vi "BinAvgSub3.vi"(6 "X ref array":dbl[](array[numeric]), 7 "Extend to 0":bool, 9 "Bin size":dbl, 10 "X coumn index":i32, 11 "Data in":dbl[][](array[numeric])) -> (3 "Binned data":dbl[][](array[numeric]) format="%#_10g")   [LabVIEW 2018]
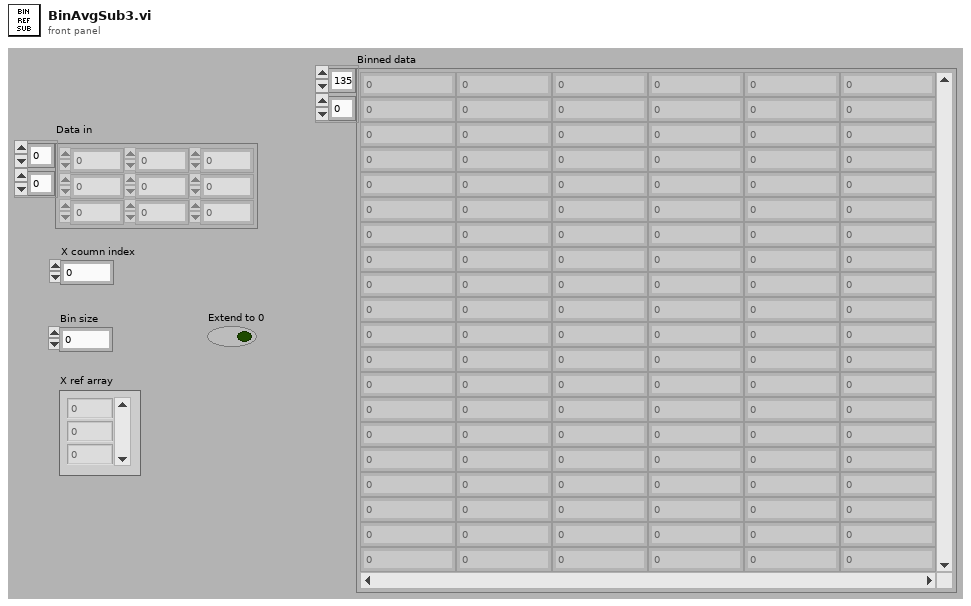
[diagram p1: front panel]
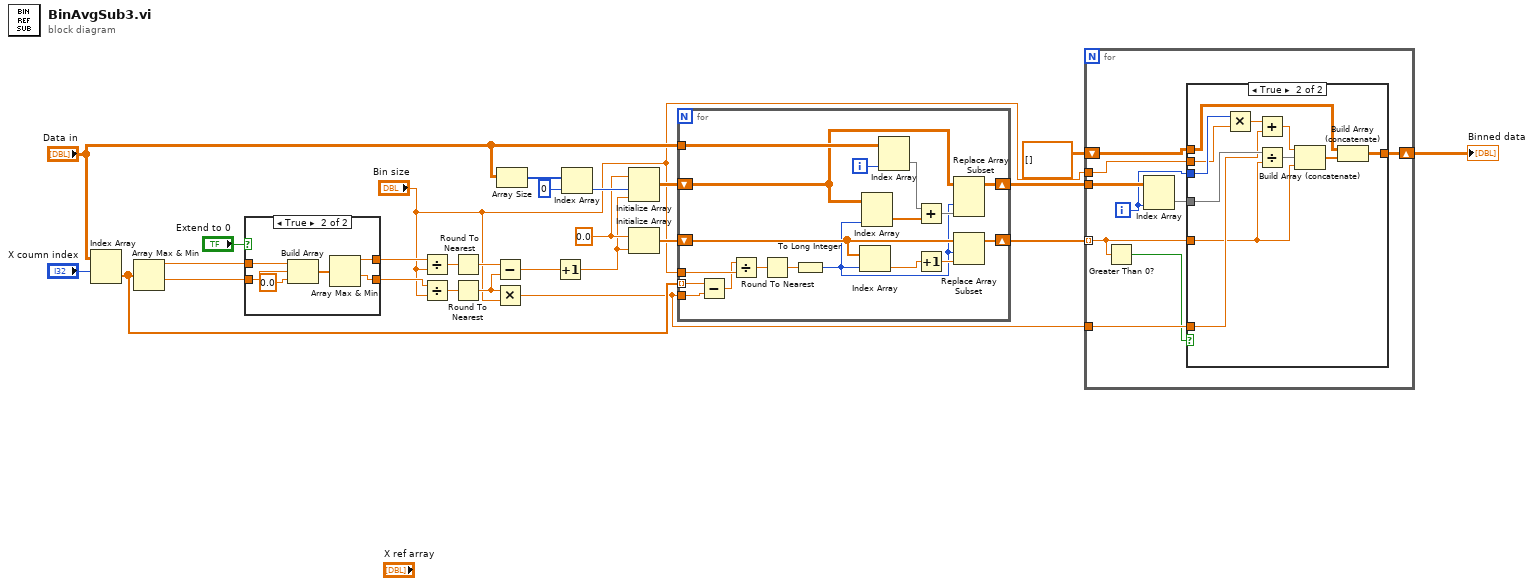
[diagram p0: block diagram]
diagram:
  w13 = 0.0 ("element")
  n1 = Index Array(array="Data in", index (row)="X coumn index") -> (element=w16:dbl[])  [unwired: 1 in]
  n2 = Array Max & Min(array=w16) -> (max value=w23:dbl, min value=w22:dbl)  [unwired: 2 out]
  n3 = case shown="True" "Extend to 0" {
    tunnel: w23 -> [w28 w34]
    tunnel: w22 -> [w27 w33]
    tunnel: [w28 w30] -> w20
    tunnel: [w27 w29] -> w21
    frame False {
    }
    frame True {
      n4 = Build Array(w34, w33, 0.0 ("element")) -> (w31:dbl[])
      n5 = Array Max & Min(array=w31) -> (max value=w30:dbl, min value=w29:dbl)  [unwired: 2 out]
    }
  }
  n6 = Divide(x=w20, y="Bin size") -> (x/y=w19:dbl)
  n7 = Divide(x=w21, y="Bin size") -> (x/y=w18:dbl)
  n8 = Round To Nearest(number=w19) -> (nearest integer value=w17:dbl)
  n9 = Round To Nearest(number=w18) -> (nearest integer value=w10:dbl)
  n10 = Subtract(x=w17, y=w10) -> (x-y=w12:dbl)
  n11 = Multiply(x=w10, y="Bin size") -> (x*y=w7:dbl)
  n12 = Array Size(array="Data in") -> (size(s)=w26:i32[])
  n13 = Increment(x=w12) -> (x+1=w5:dbl)
  n14 = Index Array(array=w26, index=0) -> (element=w14:i32)
  n15 = Initialize Array(w13, w14, w5) -> (w15:dbl[][])
  n16 = Initialize Array(w13, w5) -> (w11:dbl[])
  n17 = for {
    tunnel: w16 -> [w39] mode=indexing
    shift-right: [w46] -> w4
    shift-left: w15 -> [w47]
    tunnel: "Data in" -> [w52]
    tunnel: "Bin size" -> [w51]
    tunnel: w7 -> [w38]
    shift-right: [w45] -> w9
    shift-left: w11 -> [w44]
    i -> [w36]
    n18 = Subtract(x=w39, y=w38) -> (x-y=w40:dbl)
    n19 = Divide(x=w40, y=w51) -> (x/y=w50:dbl)
    n20 = Round To Nearest(number=w50) -> (nearest integer value=w37:dbl)
    n21 = To Long Integer(number=w37) -> (32bit integer=w35:i32)
    n22 = Index Array(array=w44, index=w35) -> (element=w48:dbl)
    n23 = Index Array(array=w47, index (col)=w35) -> (element=w42:dbl[])  [unwired: 1 in]
    n24 = Index Array(array=w52, index (col)=w36) -> (element=w49:dbl[])  [unwired: 1 in]
    n25 = Add(x=w49, y=w42) -> (x+y=w41:dbl[])
    n26 = Increment(x=w48) -> (x+1=w43:dbl)
    n27 = Replace Array Subset(array=w47, new element=w41, index (col)=w35) -> (w46:dbl[][])  [unwired: 1 in]
    n28 = Replace Array Subset(array=w44, new element=w43, index=w35) -> (w45:dbl[])
  }
  n29 = for {
    tunnel: w9 -> [w54] mode=indexing
    tunnel: "Bin size" -> [w60]
    tunnel: w7 -> [w59]
    shift-right: [w57] -> w2
    shift-left: dbl[][] [] -> [w56]
    tunnel: w4 -> [w58]
    i -> [w53]
    n30 = Greater Than 0?(x=w54) -> (x > 0?=w55:bool)
    n31 = Index Array(array=w58, index (col)=w53) -> (element=w61:dbl[])  [unwired: 1 in]
    n32 = case shown="True" w55 {
      tunnel: w61 -> [_ w73]
      tunnel: w53 -> [_ w72]
      tunnel: w60 -> [_ w71]
      tunnel: w59 -> [_ w70]
      tunnel: w54 -> [_ w66]
      tunnel: [w62 w65] -> w57
      tunnel: w56 -> [w62 w63]
      frame False {
      }
      frame True {
        n33 = Multiply(x=w72, y=w71) -> (x*y=w69:dbl)
        n34 = Add(x=w69, y=w70) -> (x+y=w68:dbl)
        n35 = Divide(x=w73, y=w66) -> (x/y=w67:dbl[])
        n36 = Build Array (concatenate)(w68, w67, w66) -> (w64:dbl[])
        n37 = Build Array (concatenate)(w63, w64) -> (w65:dbl[][])
      }
    }
  }
  "Binned data" <- w2
